vi "Enclose in Structure - Remove AC Nodes in Wires.vi"(8 "error in":errorcluster, 11 "Always Copy Nodes":refnum<vi>[](array[refnum])) -> (0 "error out":errorcluster)   [LabVIEW 2020]
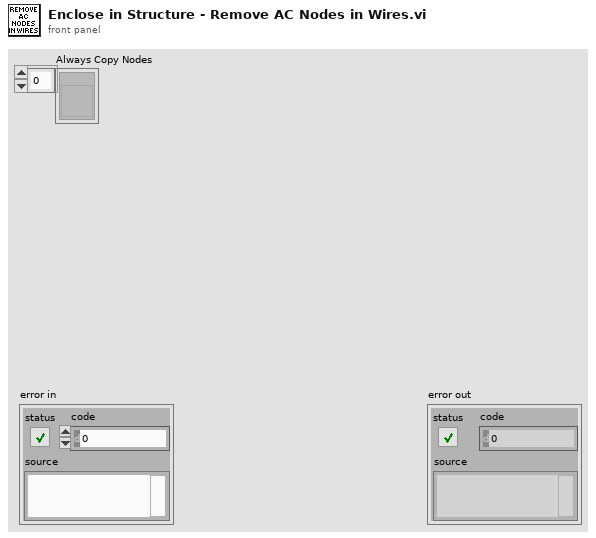
[diagram p1: front panel]
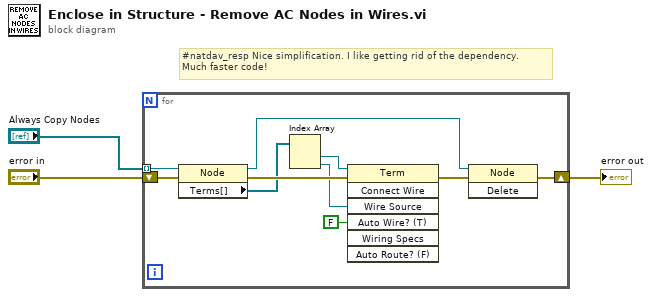
[diagram p0: block diagram]
diagram:
  # "#natdav_resp Nice simplification. I like getting rid of the dependency.\nMuch faster code!"
  n1 = for {
    tunnel: "Always Copy Nodes" -> [w10] mode=indexing
    shift-right: [w12] -> w2
    shift-left: "error in" -> [w11]
    n2 = property class="Node"(reference=w10, error in=w11) -> (reference out=w4:refnum<vi>, error out=w13:errorcluster, "Terms[]"=w9:refnum<vi>[])
    n3 = Index Array(array=w9) -> (element #1=w7:refnum<vi>, element #2=w8:refnum<vi>)  [unwired: 2 in]
    n4 = invoke class="Term" method="Connect Wire"(reference=w7, error in=w13, "Wire Source"=w8, "Auto Wire? (T)"=FALSE) -> (error out=w6:errorcluster)  [unwired: 3 in, 6 out]
    n5 = invoke class="Node" method="Delete"(reference=w4, error in=w6) -> (error out=w12:errorcluster)  [unwired: 1 in, 2 out]
  }
  "error out" <- w2
